vi "SubVI_ReadMatS_002.vi"(11 "1-bit pixmap   in":bool[][](array[boolean])) -> ()   [LabVIEW 2018]
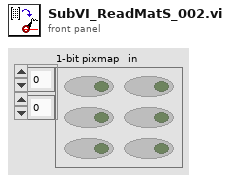
[diagram p1: front panel]
types:
  T1 = cluster{"[0]":i32, "[1]":i32, "[2]":i32, "[3]":i32, "[4]":i32, "[5]":i32, "[6]":i32, "[7]":i32, "[8]":i32}
  T2 = cluster{"[0]":dbl, "[1]":dbl, "[2]":dbl, "[3]":dbl, "[4]":dbl, "[5]":dbl, "[6]":dbl, "[7]":dbl, "[8]":dbl}
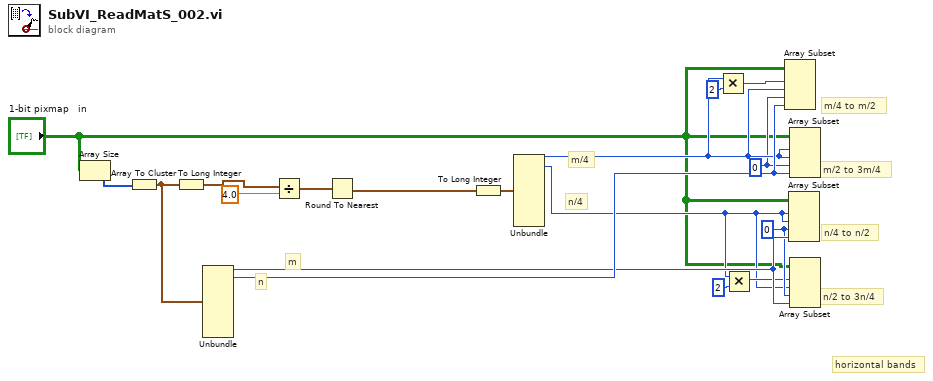
[diagram p0: block diagram]
diagram:
  w6 = 0 ("index")
  w5 = 0 ("index")
  # "n/2 to 3n/4"
  # "n/4 to n/2"
  # "m/2 to 3m/4"
  # "m/4 to m/2"
  # "horizontal bands"
  # "m"
  # "n/4"
  # "m/4"
  # "n"
  n1 = Array Size(array="1-bit pixmap   in") -> (size(s)=w17:i32[])
  n2 = Array To Cluster(array=w17) -> (cluster=w16:T1)
  n3 = To Long Integer(number=w16) -> (32bit integer=w15:T1)
  n4 = Unbundle(w16) -> ("[0]"=w7:i32, "[1]"=w11:i32)  [unwired: 7 out]
  n5 = Divide(x=w15, y=4.0) -> (x/y=w14:T2)
  n6 = Round To Nearest(number=w14) -> (nearest integer value=w13:T2)
  n7 = To Long Integer(number=w13) -> (32bit integer=w12:T1)
  n8 = Unbundle(w12) -> ("[0]"=w8:i32, "[1]"=w2:i32)  [unwired: 7 out]
  n9 = Multiply(x=w8, y=2) -> (x*y=w9:i32)
  n10 = Multiply(x=w2, y=2) -> (x*y=w3:i32)
  n11 = Array Subset(array="1-bit pixmap   in", index (row)=w9, length (row)=w8, index (col)=w5, length (col)=w11) -> ()  [unwired: 1 out]
  n12 = Array Subset(array="1-bit pixmap   in", index (row)=w2, length (row)=w2, index (col)=w6, length (col)=w7) -> ()  [unwired: 1 out]
  n13 = Array Subset(array="1-bit pixmap   in", index (row)=w8, length (row)=w8, index (col)=w5, length (col)=w11) -> ()  [unwired: 1 out]
  n14 = Array Subset(array="1-bit pixmap   in", index (row)=w3, length (row)=w2, index (col)=w6, length (col)=w7) -> ()  [unwired: 1 out]
